vi "array to degrees (SubVI).vi"(1 "acc scale":dbl=1280.0, 2 "gyro scale":dbl=8.75 format="%#_13g", 3 "all rows in in":i64[][](array[numeric])) -> (0 "Array":dbl[][](array[numeric]))   [LabVIEW 2013]
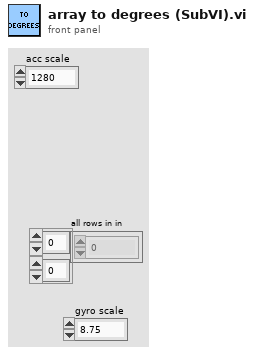
[diagram p1: front panel]
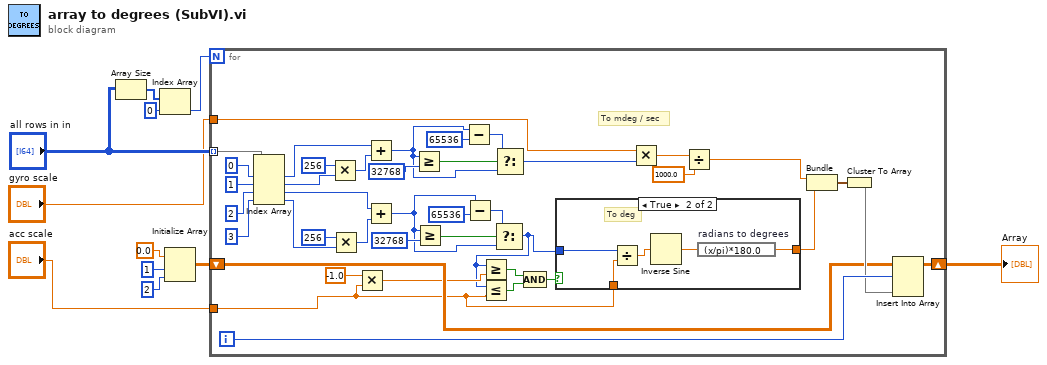
[diagram p0: block diagram]
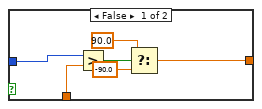
[diagram p2: hidden frame]
diagram:
  n1 = Array Size(array="all rows in in") -> (size(s)=w4:i32[])
  n2 = Index Array(array=w4, index=0) -> (element=w5:i32)
  n3 = Initialize Array(0.0 ("element"), 1 ("dimension size"), 2 ("dimension size")) -> (w10:dbl[][])
  n4 = for {
    N: w5 -> [_]
    tunnel: "all rows in in" -> [w52] mode=indexing
    shift-right: [w29] -> w11
    shift-left: w10 -> [w20]
    tunnel: "gyro scale" -> [w21]
    tunnel: "acc scale" -> [w13]
    i -> [w30]
    # "To mdeg / sec"
    n5 = Index Array(array=w52, index #1=0 ("index"), index #2=1 ("index"), index #3=2 ("index"), index #4=3 ("index")) -> (element #1=w44:i64, element #2=w47:i64, element #3=w41:i64, element #4=w43:i64)
    n6 = Multiply(x=i64 256, y=w47) -> (x*y=w45:i64)
    n7 = Multiply(x=i64 256, y=w43) -> (x*y=w40:i64)
    n8 = Multiply(x=-1.0, y=w13) -> (x*y=w15:dbl)
    n9 = Add(x=w44, y=w45) -> (x+y=w32:i64)
    n10 = Add(x=w41, y=w40) -> (x+y=w16:i64)
    n11 = Greater Or Equal?(x=w32, y=32768) -> (x >= y?=w38:bool)
    n12 = Greater Or Equal?(x=w16, y=32768) -> (x >= y?=w36:bool)
    n13 = Subtract(x=w32, y=65536) -> (x-y=w31:i64)
    n14 = Subtract(x=w16, y=65536) -> (x-y=w34:i64)
    n15 = Select(t=w34, s=w36, f=w16) -> (s? t:f=w12:i64)
    n16 = Greater Or Equal?(x=w12, y=w15) -> (x >= y?=w18:bool)
    n17 = Less Or Equal?(x=w12, y=w13) -> (x <= y?=w17:bool)
    n18 = Select(t=w31, s=w38, f=w32) -> (s? t:f=w28:i64)
    n19 = Compound Arithmetic op=AND(w18, w17) -> (w14:bool)
    n20 = case shown="True" w14 {
      tunnel: w12 -> [w56 w63]
      tunnel: [w53 w62] -> w23
      tunnel: w13 -> [w57 w59]
      frame False {
        n21 = Greater?(x=w56, y=w57) -> (0:w58:bool)
        n22 = Select(t=90.0, s=w58, f=-90.0) -> (s? t:f=w53:dbl)
      }
      frame True {
        # "To deg"
        n23 = Divide(x=w63, y=w59) -> (x/y=w61:dbl)
        n24 = Inverse Sine(1:w61) -> (0:w60:dbl)
        n25 = expression code="(x/pi)*180.0" "radians to degrees"(w60) -> (w62:dbl)
      }
    }
    n26 = Multiply(x=w21, y=w28) -> (x*y=w27:dbl)
    n27 = Divide(x=w27, y=1000.0) -> (x/y=w25:dbl)
    n28 = Bundle(w25, "f"=w23) -> (w22:cluster{dbl, "f":dbl})  [unwired: 1 in]
    n29 = Cluster To Array(cluster=w22) -> (array=w24:dbl[])
    n30 = Insert Into Array(array=w20, index (row)=w30, new element=w24) -> (w29:dbl[][])  [unwired: 1 in]
  }
  "Array" <- w11
